vi "InsertDeleteRows.vi"(0 "Start Row":i32, 1 "Col Array Ref in":refnum<vi>, 2 "Table History ref":refnum<vi>, 5 "sel size (1)":i32=1, 7 "# times (1)":i32=1, 9 "Table CtlRef In":refnum<vi>, 11 "error in (no error)":errorcluster, 12 "Layout Ring Refnum":refnum<vi>, 13 "Mode Col Index":i32) -> (4 "Col Array Ref out":refnum<vi>, 10 "Table CtlRef Out":refnum<vi>, 15 "error out":errorcluster)   [LabVIEW 2013]
doc: "Inserting and deleting entire row(s) affects the formatting of most of the table. Therefore, this utility calls \"format all\" after modifying the string array value of the table. For \"# times\" > 0, the \"sel size\" rows beginning with \"start row\" are inserted \"# times.\" With \"# times\" < 0, \"sel size\" x \"# times\" rows are deleted beginning with the start row. Also, the undo/redo table history is updated if \"Table History ref\" is wired.\n\nPerformance could be improved by calling a more precise formatting function which compares the present table to the history instead of blanket formatting the entire table."
uses:
  TypeDefs/TableHistory.ctl
  TypeDefs/TableArray.ctl
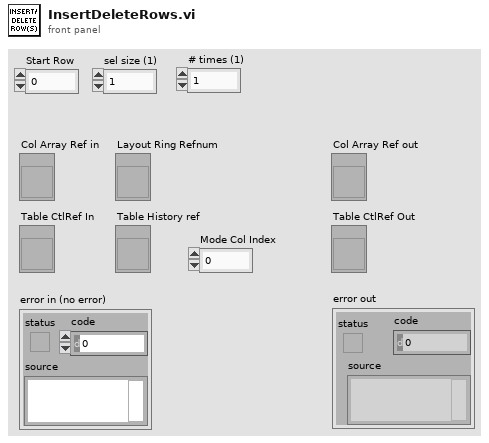
[diagram p1: front panel]
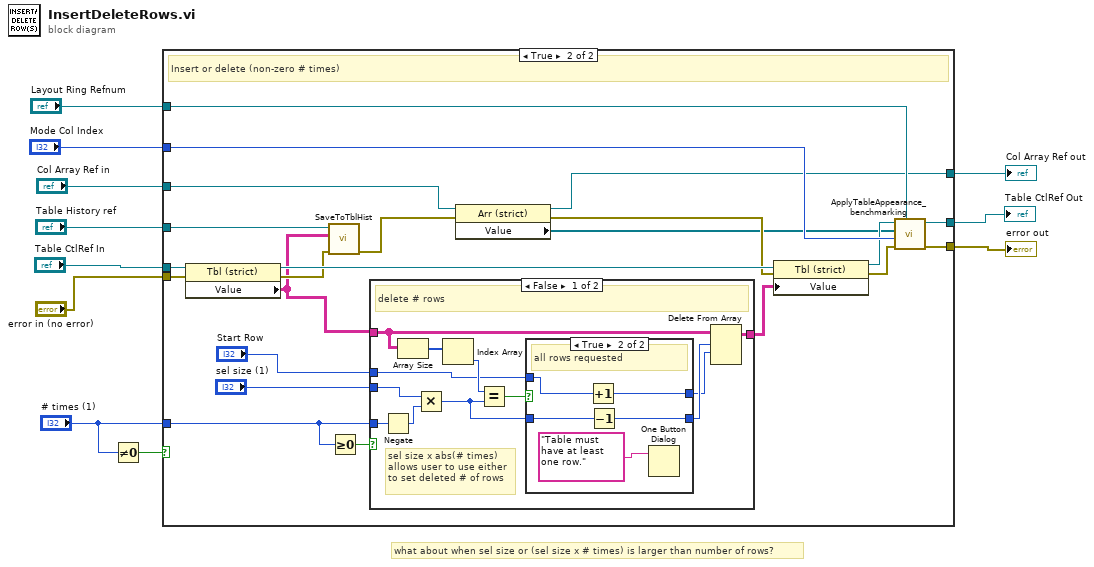
[diagram p0: block diagram]
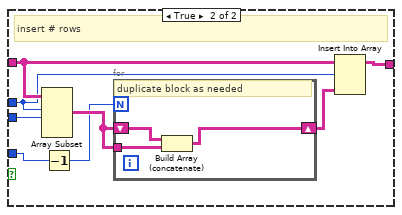
[diagram p4: hidden frame]
diagram:
  # "what about when sel size or (sel size x # times) is larger than number of rows?"
  n1 = Not Equal To 0?(x="# times (1)") -> (x != 0?=w1:bool)
  n2 = case shown="True" w1 {
    tunnel: "Table CtlRef In" -> [w13 w36]
    tunnel: "error in (no error)" -> [w12 w35]
    tunnel: "Table History ref" -> [_ w30]
    tunnel: [w12 w26] -> w8
    tunnel: "Mode Col Index" -> [_ w25]
    tunnel: [w13 w23] -> w6
    tunnel: "Layout Ring Refnum" -> [_ w22]
    tunnel: "Col Array Ref in" -> [w14 w21]
    tunnel: [w14 w20] -> w3
    tunnel: "# times (1)" -> [_ w15]
    frame False {
      # "# times = 0: indicates do nothing (e.g. user cancelled delete)"
    }
    frame True {
      # "Insert or delete (non-zero # times)"
      n3 = property class="Tbl (strict)"(reference=w36, error in=w35) -> (reference out=w33:refnum<vi>, error out=w31:errorcluster, "Value"=w29:string[][])
      n4 = call "SaveToTblHist.vi"("error in (no error)"=w31, "OldTable (reset)"=w29, "Table History ref"=w30) -> ("error out"=w19:errorcluster)  [unwired: 8 in]
      n5 = Greater Or Equal To 0?(x=w15) -> (x >= 0?=w16:bool)
      n6 = case shown="False" w16 {
        tunnel: [w48 w63] -> w34
        tunnel: "sel size (1)" -> [w47 w61]
        tunnel: w29 -> [w44 w62]
        tunnel: "Start Row" -> [w40 w57]
        tunnel: w15 -> [w46 w59]
        frame False {
          # "sel size x abs(# times)\nallows user to use either\nto set deleted # of rows"
          # "delete # rows"
          n7 = Negate(x=w46) -> (-x=w45:i32)
          n8 = Array Size(array=w44) -> (size(s)=w43:i32[])
          n9 = Multiply(x=w47, y=w45) -> (x*y=w39:i32)
          n10 = Index Array(array=w43) -> (element=w42:i32)  [unwired: 1 in]
          n11 = Equal?(x=w42, y=w39) -> (x = y?=w41:bool)
          n12 = case shown="True" w41 {
            tunnel: w40 -> [w50 w55]
            tunnel: w39 -> [w49 w54]
            tunnel: [w50 w53] -> w37
            tunnel: [w49 w52] -> w38
            frame False {
              # "# rows OK"
            }
            frame True {
              # "all rows requested"
              n13 = Increment(x=w55) -> (x+1=w53:i32)
              n14 = Decrement(x=w54) -> (x-1=w52:i32)
              n15 = One Button Dialog(message="Table must have at least one row.") -> ()  [unwired: 1 in, 1 out]
            }
          }
          n16 = Delete From Array(array=w44, length=w38, index (row)=w37) -> (array with subset deleted=w48:string[][])  [unwired: 1 in, 1 out]
        }
        frame True {
          # "insert # rows"
          n17 = Array Subset(array=w62, index (row)=w57, length (row)=w61) -> (w60:string[][])  [unwired: 2 in]
          n18 = Decrement(x=w59) -> (x-1=w58:i32)
          n19 = for {
            N: w58 -> [_]
            shift-right: [w64] -> w56
            shift-left: w60 -> [w66]
            tunnel: w60 -> [w65]
            # "duplicate block as needed"
            n20 = Build Array (concatenate)(w66, w65) -> (w64:string[][])
          }
          n21 = Insert Into Array(array=w62, index (row)=w57, new element=w56) -> (w63:string[][])  [unwired: 1 in]
        }
      }
      n22 = property class="Arr (strict)"(reference=w21, error in=w19) -> (reference out=w20:refnum<vi>, error out=w18:errorcluster, "Value"=w17:refnum<class "Column.lvclass">[])
      n23 = property class="Tbl (strict)"(reference=w33, error in=w18, "Value"=w34) -> (reference out=w24:refnum<vi>, error out=w27:errorcluster)
      n24 = call "ApplyTableAppearance_benchmarking.vi"("Layout Ring Ref"=w22, "error in (no error)"=w27, "Mode Index"=w25, "Col Array in"=w17, "Table Ref in"=w24) -> ("error out"=w26:errorcluster, "Table Ref out"=w23:refnum<vi>)  [unwired: 5 in]
    }
  }
  "error out" <- w8
  "Table CtlRef Out" <- w6
  "Col Array Ref out" <- w3
